vi "parse_int64.vi"   [LabVIEW 2010]
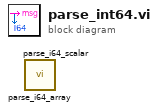
[diagram p0: block diagram]
diagram:
  n1 = call <userlib>:"parse_i64_array.vi"() -> ()  [unwired: 5 in, 3 out]
  n2 = call <userlib>:"parse_i64_scalar.vi"() -> ()  [unwired: 5 in, 3 out]
